vi "Write_Error_Msg.vi"(8 "error in (no error)":errorcluster) -> (3 "concatenated string":string)   [LabVIEW 2014, in "Manipulator.lvclass"]
uses:
  Manipulator.lvclass
  <vilib>/Utility/sysdir.llb/System Directory Type.ctl
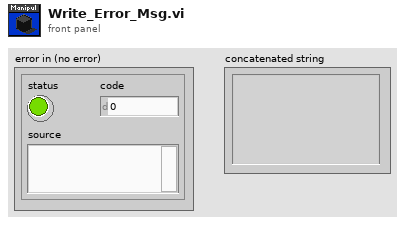
[diagram p1: front panel]
types:
  T1 = enum16{"open", "replace", "create", "open or create", "replace or create", "replace or create with confirmation"}
  T2 = typedef "System Directory Type.ctl" = i32
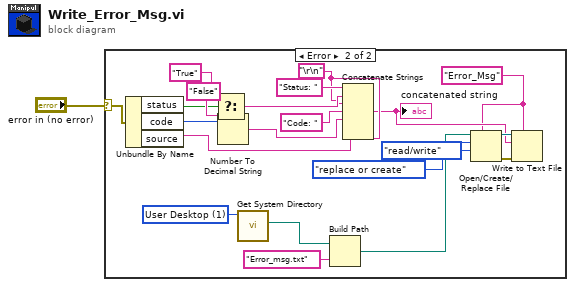
[diagram p0: block diagram]
diagram:
  n1 = case shown="Error" "error in (no error)" {
    selector: "error in (no error)" -> [_ w22]
    frame No Error {
    }
    frame Error {
      w9 = "Error_Msg" ("prompt (Choose or enter file path)")
      w13 = T2 1 items=["User Home"=0, "User Desktop"=1, "User Documents"=2, "User Application Data"=3, "User Preferences"=4, "User Temporary"=5, "Public Documents"=6, "Public Application Data"=7, "Public Preferences"=8, "Public Cache"=13, "System Core Libraries"=9, "System Installed Libraries"=10, "Application Files"=11, "Boot Volume Root"=12] ("system directory type")
      w15 = "\r\n"
      n2 = Unbundle By Name(w22) -> ("status"=w5:bool, "code"=w4:i32, "source"=w3:string)
      n3 = Select(t="True", s=w5, f="False") -> (s? t:f=w18:string)
      n4 = Number To Decimal String(number=w4) -> (decimal integer string=w16:string)  [unwired: 1 in]
      n5 = call <vilib>:"Get System Directory.vi"("system directory type"=w13) -> ("system directory"=w8:path)  [unwired: 10 in]
      n6 = Build Path(base path=w8, name or relative path="Error_msg.txt") -> (appended path=w2:path)
      n7 = Concatenate Strings("Status: ", w18, w15, "Code: ", w16, w15, w3) -> (w10:string)
      "concatenated string" <- w10
      n8 = Open/Create/Replace File(file path (use dialog)=w2, prompt=w9, operation (0:open)=T1."replace or create", access (0:read/write)=enum16{"read/write", "read-only", "write-only"}."read/write") -> (refnum out=w11:refnum<file>, error out=w12:errorcluster)  [unwired: 2 in, 1 out]
      n9 = Write to Text File(prompt (Choose or enter file path)=w9, file (use dialog)=w11, text=w10, error in=w12) -> ()  [unwired: 3 out]
    }
  }
